vi "Read (Single _mod).vi"(0 "VISA resource name":refnum<visa-resource-name>, 1 "Channel (0: Channel 1)":u16(ring) items=["Channel 1", "Channel 2", "Channel 3", "Channel 4"], 2 "Measurement Function (0: Voltage Vpp) 2":u16(ring) items=["Voltage Vpp", "Voltage Max", "Voltage Min", "Amplitude", "Voltage TOP", "Voltage Base", "Voltage Average", "Voltage RMS", "Overshoot", "Preshoot", "Frequency", "Rise Time", "Fall Time", "Period", "Positive Width", "Negative Width", "Positive Duty", "Negative Duty"], 3 "Measurement Function (0: Voltage Vpp)":u16(ring) items=["Voltage Vpp", "Voltage Max", "Voltage Min", "Amplitude", "Voltage TOP", "Voltage Base", "Voltage Average", "Voltage RMS", "Overshoot", "Preshoot", "Frequency", "Rise Time", "Fall Time", "Period", "Positive Width", "Negative Width", "Positive Duty", "Negative Duty"], 4 "Timeout (10000 ms)":u32=10000, 5 "error in (no error)":errorcluster) -> (14 "VISA resource name out":refnum<visa-resource-name>, 15 "M2":dbl, 16 "M1":dbl, 17 "Waveform Data":waveform(dbl)(graph), 19 "error out":errorcluster)   [LabVIEW 2018]
doc: "Initiates an acquisition on all channels that you enabled with the Configure Channel VI. The VI waits for the acquisition to complete and returns the waveform for the <B>Source Channel</B> you specified. If the oscilloscope did not complete the acquisition within the time period you specify with the <B>Timeout</B> control, the VI returns a timeout error. A common cause for a timeout error is the acquisition was not triggered. For example, the trigger level is out of range of the waveform."
uses:
  <instrlib>/RIGOL DS1000 Series/RIGOL DS1000 Series.lvlib
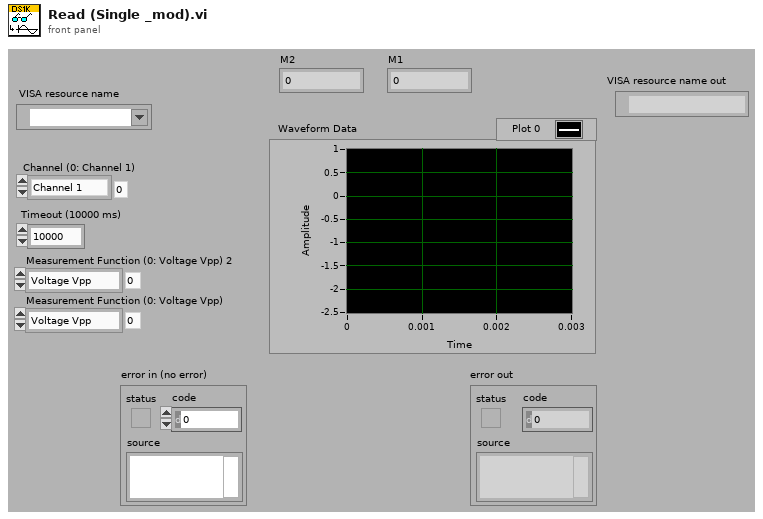
[diagram p1: front panel]
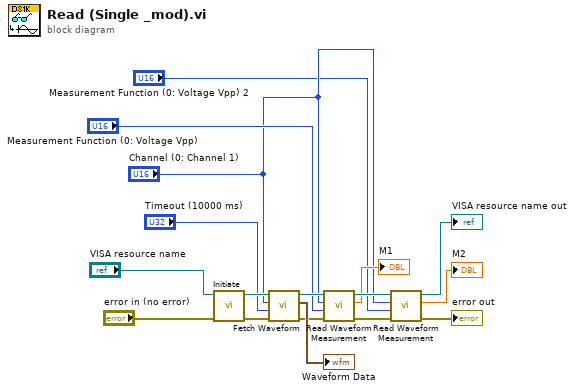
[diagram p0: block diagram]
diagram:
  n1 = call <instrlib>:"Initiate.vi"("error in (no error)"="error in (no error)", "VISA resource name"="VISA resource name") -> ("error out"=w14:errorcluster, "VISA resource name out"=w15:refnum<visa-resource-name>)  [unwired: 8 out]
  n2 = call <instrlib>:"Fetch Waveform.vi"("error in (no error)"=w14, "Timeout (10000 ms)"="Timeout (10000 ms)", "Channel (0: Channel 1)"="Channel (0: Channel 1)", "VISA resource name"=w15) -> ("error out"=w7:errorcluster, "Waveform Data"=→"Waveform Data":waveform(dbl), "VISA resource name out"=w11:refnum<visa-resource-name>)  [unwired: 5 out]
  n3 = call <instrlib>:"Read Waveform Measurement.vi"("error in (no error)"=w7, "Measurement Function (0: Voltage Vpp)"="Measurement Function (0: Voltage Vpp)", "Source (0: Channel 1)"="Channel (0: Channel 1)", "VISA resource name"=w11) -> ("error out"=w3:errorcluster, "Measured Value"=→"M1":dbl, "VISA resource name out"=w10:refnum<visa-resource-name>)  [unwired: 5 in]
  n4 = call <instrlib>:"Read Waveform Measurement.vi"("error in (no error)"=w3, "Measurement Function (0: Voltage Vpp)"="Measurement Function (0: Voltage Vpp) 2", "Source (0: Channel 1)"="Channel (0: Channel 1)", "VISA resource name"=w10) -> ("error out"=→"error out":errorcluster, "Measured Value"=→"M2":dbl, "VISA resource name out"=→"VISA resource name out":refnum<visa-resource-name>)  [unwired: 5 in]
